vi "2. Main.vi"() -> ()   [LabVIEW 2013]
uses:
  src/LabVIEW/LQ Core/QSize.ctl
  src/LabVIEW/Qt Widgets/QBoxLayout/Direction.ctl
  src/LabVIEW/Qt Widgets/QWidget/resize.vi
  src/LabVIEW/Qt Widgets/QWidget/setVisible.vi
  src/LabVIEW/LQ Core/LQCoreEngine/LQCoreEngine.lvclass
  src/LabVIEW/Qt Widgets/QLCDNumber/QLCDNumber.lvclass
  src/LabVIEW/Qwt/QwtSlider/QwtSlider.lvclass
  src/LabVIEW/Qt Widgets/QWidget/QWidget.lvclass
  src/LabVIEW/Qt Widgets/QBoxLayout/QBoxLayout.lvclass
panel:
  in  "Stop Button":bool
  # "Prerequisite knowledge/experience\n- Example 1. Constructing and Using a Widget\n\n\nDescription\nLayouts provide a way to intelligently allocate space to multiple widgets within the same window.\nThis space allocation is dynamic: When you resize the window, all widgets in it get resized accordingly.\n\nThis example shows two widgets in a vertical QBoxLayout, one above the other. Other available layouts\nare QGridLayout and QFormLayout.\n\n\nInstructions\n1. Run this VI and watch the widgets.\n2. Use your mouse to resize the top-level widget. (Notice that the LCD resizes both horizontally and\n    vertically, while the slider only resizes horizontally)\n3. Click \"Stop\".\n\n\nShowcase\n- Dynamically resizing layouts"
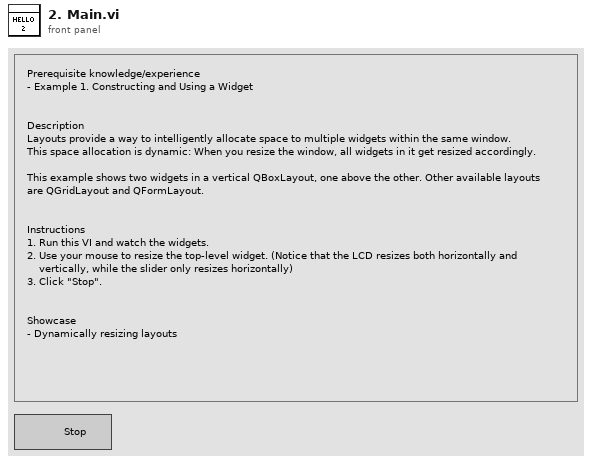
[diagram p1: front panel]
types:
  T1 = typedef "QBoxLayout.lvclass/Direction.ctl" = i32
  T2 = typedef "QSize.ctl" = cluster{"width":i32, "height":i32}
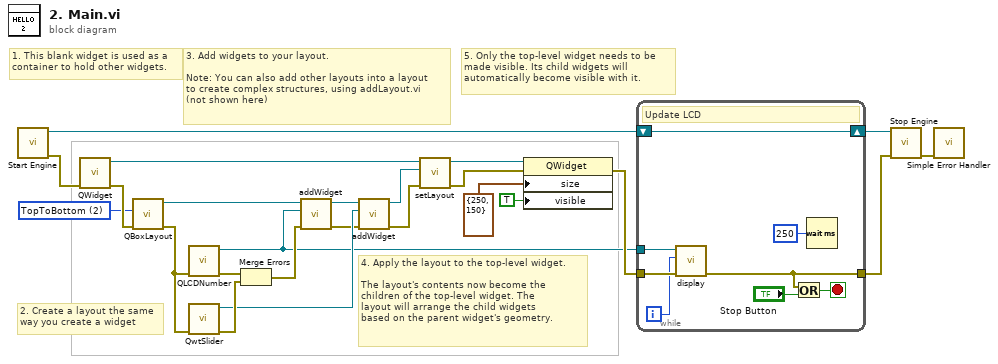
[diagram p0: block diagram]
diagram:
  w1 = T1 2 items=["LeftToRight", "RightToLeft", "TopToBottom", "BottomToTop"] ("direction")
  # "2. Create a layout the same\nway you create a widget"
  # "5. Only the top-level widget needs to be\nmade visible. Its child widgets will\nautomatically become visible with it."
  # "4. Apply the layout to the top-level widget.\n\nThe layout's contents now become the\nchildren of the top-level widget. The\nlayout will arrange the child widgets\nbased on the parent widget's geometry."
  # "3. Add widgets to your layout.\n\nNote: You can also add other layouts into a layout\nto create complex structures, using addLayout.vi\n(not shown here)"
  # "1. This blank widget is used as a\ncontainer to hold other widgets."
  n1 = call "Start Engine.vi"() -> ("Error Out"=w17:errorcluster, "New Engine"=w22:refnum<class "LQCoreEngine.lvclass">)  [unwired: 10 in]
  n2 = call "QWidget.vi"("Error In"=w17) -> ("Error Out"=w16:errorcluster, "New QWidget"=w8:refnum<class "QWidget.lvclass">)  [unwired: 9 in]
  n3 = call "QBoxLayout.vi"("Error In"=w16, "direction"=w1) -> ("Error Out"=w15:errorcluster, "New QBoxLayout"=w14:refnum<class "QBoxLayout.lvclass">)  [unwired: 8 in]
  n4 = call "QLCDNumber.vi"("Error In"=w15) -> ("Error Out"=w12:errorcluster, "New QLCDNumber"=w3:refnum<class "QLCDNumber.lvclass">)  [unwired: 9 in]
  n5 = call "QwtSlider.vi"("Error In"=w15) -> ("Error Out"=w13:errorcluster, "New QwtSlider"=w10:refnum<class "QwtSlider.lvclass">)  [unwired: 9 in]
  n6 = Merge Errors(w12, w13) -> (w23:errorcluster)
  n7 = call "addWidget.vi"("Error In"=w23, "widget"=w3, "QBoxLayout In"=w14) -> ("Error Out"=w9:errorcluster, "QBoxLayout Out"=w11:refnum<class "QBoxLayout.lvclass">)  [unwired: 7 in]
  n8 = call "addWidget.vi"("Error In"=w9, "widget"=w10, "QBoxLayout In"=w11) -> ("Error Out"=w6:errorcluster, "QBoxLayout Out"=w7:refnum<class "QBoxLayout.lvclass">)  [unwired: 7 in]
  n9 = call "setLayout.vi"("Error In"=w6, "layout"=w7, "QWidget In"=w8) -> ("Error Out"=w4:errorcluster, "QWidget Out"=w5:refnum<class "QWidget.lvclass">)  [unwired: 7 in]
  n10 = property class="QWidget"(reference=w5, error in=w4, "size"=T2 {"width"=250, "height"=150}, "visible"=TRUE) -> (error out=w24:errorcluster)  [unwired: 1 out]
  n11 = while {
    shift-right: [w32] -> w21
    shift-left: w22 -> [w32]
    tunnel: w24 -> [w27]
    tunnel: [w26] -> w18
    tunnel: w3 -> [w28]
    i -> [w25]
    stop <- w30 stop-if-true
    # "Update LCD"
    n12 = call "display.vi"("Error In"=w27, "num"=w25, "QLCDNumber In"=w28) -> ("Error Out"=w26:errorcluster)  [unwired: 7 in, 1 out]
    n13 = Or(x=w26, y="Stop Button") -> (x .or. y?=w30:bool)
    n14 = Wait (ms)(milliseconds to wait=u32 250) -> ()  [unwired: 1 out]
  }
  n15 = call "Stop Engine.vi"("Error In"=w18, "LQCoreEngine"=w21) -> ("Error Out"=w20:errorcluster)  [unwired: 9 in]
  n16 = call <vilib>:"Simple Error Handler.vi"("error in (no error)"=w20) -> ()  [unwired: 4 in, 5 out]
